vi "Untitled 8.vi"() -> ()   [LabVIEW 2018]
uses:
  <vilib>/Modbus/subvis/Modbus API/Modbus API.lvclass/Modbus API.ctl
  <vilib>/Modbus/subvis/Transmission Data Unit (ADU)/Transmission Data Unit/Transmission Data Unit.lvclass/Transmission Data Unit.ctl
  <vilib>/Modbus/master/Data Access/Unit ID/Set Unit ID Property.vi
  <vilib>/Modbus/subvis/Transmission Data Unit (ADU)/Transmission Data Unit/Data Access/Unit ID/Write Unit ID.vi
  <vilib>/Modbus/subvis/Modbus API/Read Transmission Data Unit.vi
  <vilib>/Modbus/subvis/Modbus API/Write Transmission Data Unit.vi
  <vilib>/Modbus/master/Modbus Master.lvclass
  C:/Program Files/National Instruments/LabVIEW 2018/vi.lib/Modbus/subvis/Modbus API/Modbus API.lvclass
  <vilib>/Modbus/master/Create Master Instance (TCP).vi
  <vilib>/Modbus/subvis/Transmission Data Unit (ADU)/Transmission Data Unit/Transmission Data Unit.lvclass
panel:
  out "appended array":u16[](array[numeric])
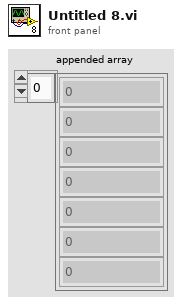
[diagram p1: front panel]
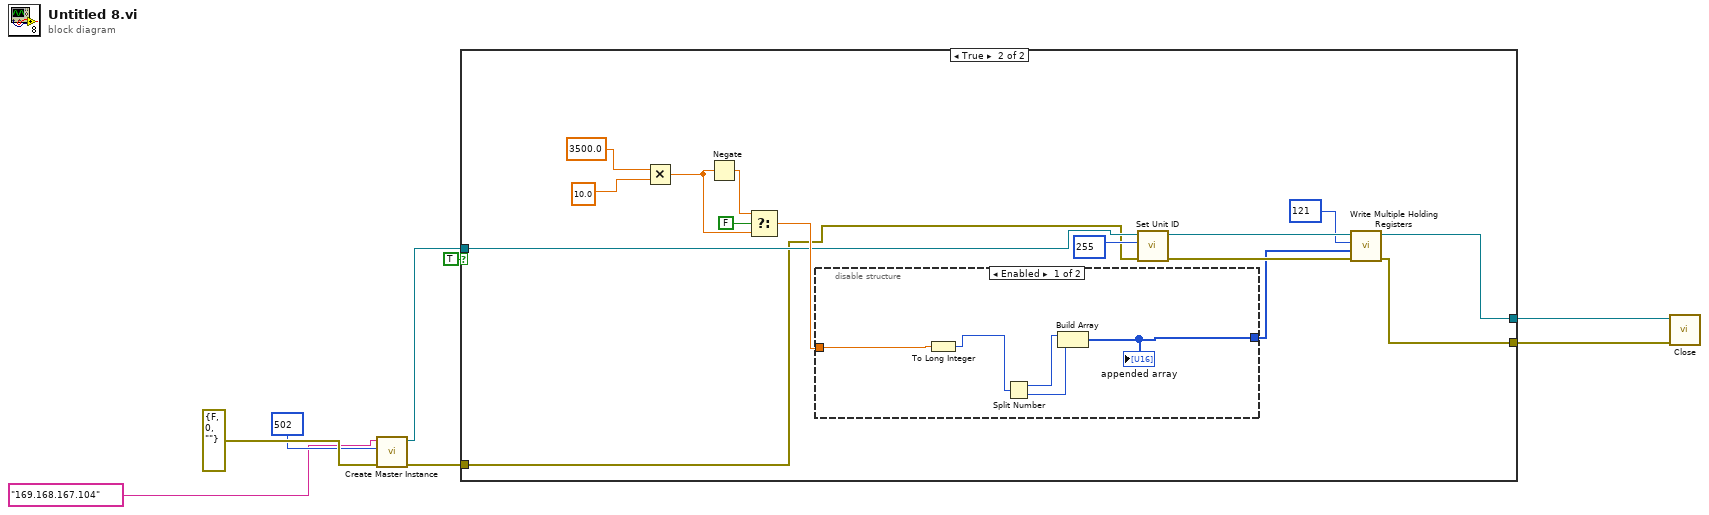
[diagram p0: block diagram]
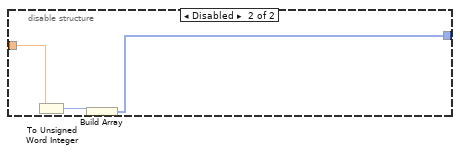
[diagram p3: hidden frame]
diagram:
  n1 = call-poly <vilib>:"Create Master Instance.vi"("error in (no error)"=errorcluster {"status"=FALSE, "code"=0, "source"=""} ("error out"), "port (502)"=u16 502, "address"="169.168.167.104") -> ("error out"=w4:errorcluster, "TCP master instance"=w5:refnum<class "Modbus Master.lvclass">)  [unwired: 7 in]
  n2 = case shown="True" TRUE {
    tunnel: w5 -> [w10 w16]
    tunnel: w4 -> [w9 w15]
    tunnel: [w10 w14] -> w3
    tunnel: [w9 w13] -> w2
    frame False {
    }
    frame True {
      n3 = Multiply(x=3500.0 ("y"), y=sgl 10.0) -> (x*y=w20:dbl)
      n4 = Negate(x=w20) -> (-x=w19:dbl)
      n5 = Select(t=w19, s=FALSE, f=w20) -> (s? t:f=w18:dbl)
      n6 = disable-structure shown="Enabled" {
        disable-tunnel: w18 -> [w29 w33]
        disable-tunnel: [w30 w31] -> w11
        frame Enabled {
          n7 = To Long Integer(number=w29) -> (32bit integer=w28:i32)
          n8 = Split Number(x=w28) -> (hi(x)=w27:u16, lo(x)=w26:u16)
          n9 = Build Array(w27, w26) -> (w30:u16[])
          "appended array" <- w30
        }
        frame Disabled {
          n10 = To Unsigned Word Integer(number=w33) -> (unsigned 16bit integer=w32:u16)
          n11 = Build Array(w32) -> (w31:u16[])
        }
      }
      n12 = call <vilib>:"Set Unit ID.vi"("error in (no error)"=w15, "unit ID"=u8 255, "Modbus master in"=w16) -> ("error out"=w22:errorcluster, "Modbus master out"=w23:refnum<class "Modbus Master.lvclass">)  [unwired: 7 in]
      n13 = call-dynamic "Write Multiple Holding Registers.vi"("error in (no error)"=w22, "holding register values"=w11, "starting address"=u16 121, "Modbus master in"=w23) -> ("error out"=w13:errorcluster, "Modbus master out"=w14:refnum<class "Modbus Master.lvclass">)  [unwired: 6 in]
    }
  }
  n14 = call-dynamic "Close.vi"("error in (no error)"=w2, "Modbus master in"=w3) -> ()  [unwired: 9 in, 1 out]
